vi "LIA Read AI and VCO Samples.vi"(8 "error in (no error)":errorcluster, 10 "samples to read":u32, 11 "fpga session in":T1) -> (0 "error out":errorcluster, 2 "VCO":dbl[](array[numeric]), 3 "AI":sgl[](array[numeric]))   [LabVIEW 2017]
uses:
  Program Files (x86)/National Instruments/LabVIEW 2017/examples/Lock-In Amplifier/lib/host/Public/fpga type.ctl
  Program Files (x86)/National Instruments/LabVIEW 2017/examples/Lock-In Amplifier/lib/host/Lock-In Amplifier Example Host.lvlib
  <vilib>/rvi/interface/nirviMethod/nirviMethod.xnode
  <instrlib>/_niInstr/Streaming/v1/Host/niInstr Streaming v1 Host.lvlib
  <instrlib>/_niInstr/Streaming/v1/Host/Public/Start Finite Stream.vi
  <vilib>/FPGAPlugInAG/Dynamic/niLvFpga_ReadFifo_Dynamic.vi
  <vilib>/rvi/errors/niLvFpgaMergeErrorWithErrorCode.vi
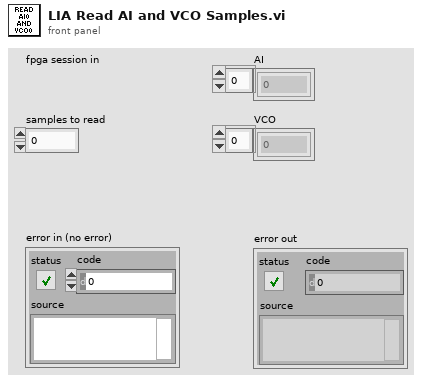
[diagram p1: front panel]
types:
  T1 = typedef "Lock-In Amplifier Example Host.lvlib/fpga type.ctl" = refnum<k20>
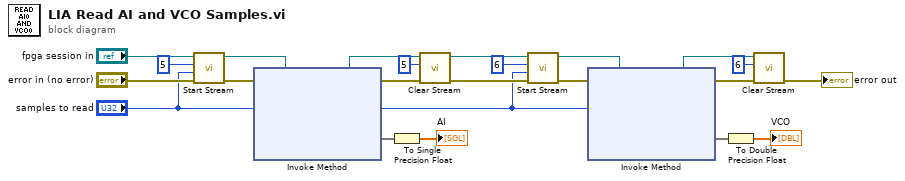
[diagram p0: block diagram]
diagram:
  n1 = call-poly <instrlib>:"Start Stream.vi"("error in (no error)"="error in (no error)", "num samples"="samples to read", "stream index"=5, "refnum in"="fpga session in") -> ("error out"=w21:errorcluster, "refnum out"=w17:T1)  [unwired: 6 in]
  n2 = xnode "Invoke Method"("FPGA VI Reference In"=w17, "error in"=w21, "Number of Elements"="samples to read") -> ("FPGA VI Reference Out"=w20:T1, "error out"=w19:errorcluster, "Data"=w16:void[])  [unwired: 1 in, 1 out]
  n3 = To Single Precision Float(number=w16) -> (single precision float=→"AI":sgl[])
  n4 = call <instrlib>:"Clear Stream.vi"("error in (no error)"=w19, "stream index"=5, "refnum in"=w20) -> ("error out"=w6:errorcluster, "refnum out"=w5:T1)  [unwired: 7 in]
  n5 = call-poly <instrlib>:"Start Stream.vi"("error in (no error)"=w6, "num samples"="samples to read", "stream index"=6, "refnum in"=w5) -> ("error out"=w12:errorcluster, "refnum out"=w8:T1)  [unwired: 6 in]
  n6 = xnode "Invoke Method"("FPGA VI Reference In"=w8, "error in"=w12, "Number of Elements"="samples to read") -> ("FPGA VI Reference Out"=w11:T1, "error out"=w10:errorcluster, "Data"=w7:void[])  [unwired: 1 in, 1 out]
  n7 = To Double Precision Float(number=w7) -> (double precision float=→"VCO":dbl[])
  n8 = call <instrlib>:"Clear Stream.vi"("error in (no error)"=w10, "stream index"=6, "refnum in"=w11) -> ("error out"=→"error out":errorcluster)  [unwired: 7 in, 1 out]
